vi "ParseDailies.vi"(8 "error in (no error)":errorcluster, 11 "file path in":path) -> (0 "error out":errorcluster, 3 "Map":map{string, dbl[]}(c390))   [LabVIEW 2019]
uses:
  <vilib>/LAVA/Robust CSV/Robust CSV.lvlib
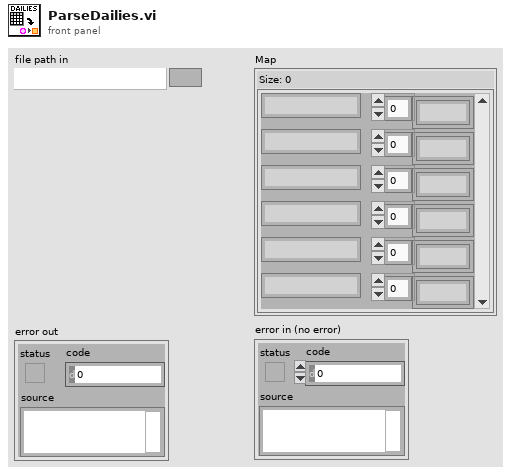
[diagram p1: front panel]
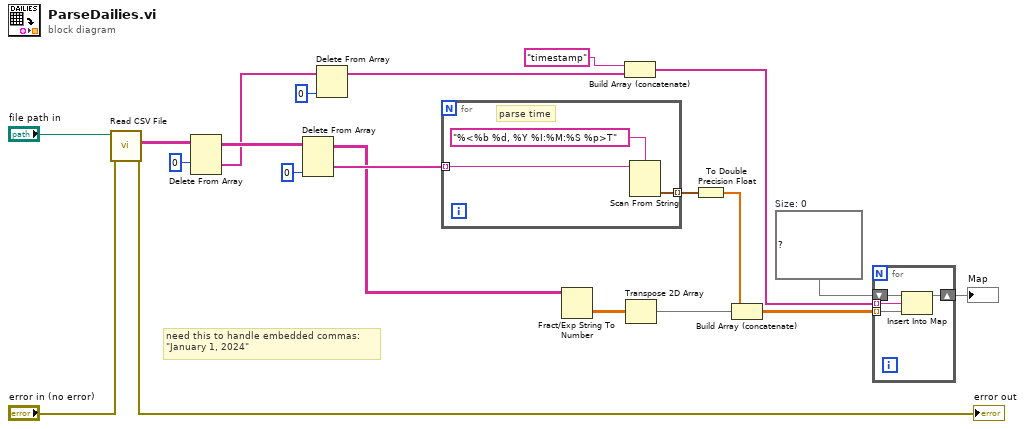
[diagram p0: block diagram]
diagram:
  w9 = map{string, dbl[]} {}  # Size: 0
  # "need this to handle embedded commas:\n\"January 1, 2024\""
  n1 = call <vilib>:"Read CSV File.vi"("error in (no error)"="error in (no error)", "file path in"="file path in") -> ("error out"=→"error out":errorcluster, "2-D array"=w20:string[][])  [unwired: 7 in, 1 out]
  n2 = Delete From Array(array=w20, index (row)=0) -> (deleted portion=w14:string[], array with subset deleted=w18:string[][])  [unwired: 2 in]
  n3 = Delete From Array(array=w18, index (col)=0 ("disabled index (col)")) -> (deleted portion=w16:string[], array with subset deleted=w15:string[][])  [unwired: 2 in]
  n4 = Delete From Array(array=w14, index=0) -> (array with subset deleted=w6:string[])  [unwired: 1 in, 1 out]
  n5 = for {
    tunnel: w16 -> [w22] mode=indexing
    tunnel: [w23] -> w8 mode=indexing
    # "parse time"
    n6 = Scan From String(format string="%<%b %d, %Y %I:%M:%S %p>T", input string=w22) -> (output 1=w23:timestamp)  [unwired: 3 in, 3 out]
  }
  n7 = Fract/Exp String To Number(string=w15) -> (number=w12:dbl[][])  [unwired: 3 in, 1 out]
  n8 = Build Array (concatenate)("timestamp", w6) -> (w2:string[])
  n9 = Transpose 2D Array(2D array=w12) -> (transposed array=w4:dbl[][])
  n10 = To Double Precision Float(number=w8) -> (double precision float=w5:dbl[])
  n11 = Build Array (concatenate)(w5, w4) -> (w3:dbl[][])
  n12 = for {
    tunnel: w3 -> [w25] mode=indexing
    tunnel: w2 -> [w28] mode=indexing
    shift-right: [w27] -> w11
    shift-left: w9 -> [w26]
    n13 = Insert Into Map(map in=w26, key=w28, value=w25) -> (map out=w27:map{string, dbl[]})  [unwired: 2 out]
  }
  "Map" <- w11
